vi "VisualizeDigitizer.vi"() -> ()   [LabVIEW 2014, in "Visualization.lvlib" / "VisualizeDigitizer.lvclass"]
uses:
  VisualizeDigitizer.lvclass
  Digitizer/DigitizerPlugins/DigitizerBaseClass/Typedefs/WfrmAttributes.ctl
  VisualizeBase/VisualizeBase_class/Requests/clUserEventType.ctl
  <vilib>/event_ctls.llb/usereventprio.ctl
  <vilib>/Utility/error.llb/Error Cluster From Error Code.vi
  <vilib>/ErrorRing/Error Ring.xnode
  VisualizeBase/VisualizeBase_class/VisualizeBase.lvclass
  <userlib>/NIST/NISTErrorLib/NISTErrorLib.lvlib
  Digitizer/DigitizerModule/DigitizerModule.lvlib
  Digitizer/DigitizerPlugins/DigitizerBaseClass/DigitizerBase.lvclass
panel:
  out "Timing":cluster{"Time Stamp":timestamp, "dt":dbl}[][](array[cluster])
  in  "btnReset":bool
  in  "btnClear":bool
  out "Attributes":T1[][](array[typedef])
  out "Waveform":waveform(dbl)[](graph)
  in  "QueName":string="DigitizerVisQue"
  out "ErrorArray":errorcluster[](array[cluster])
  in  "btnStop":bool
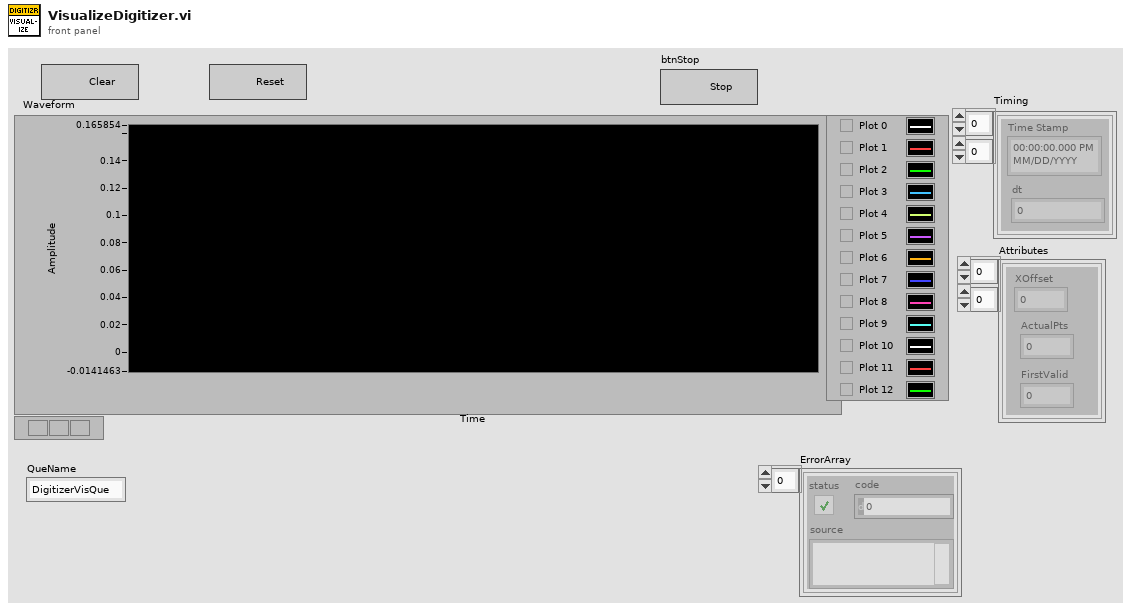
[diagram p1: front panel]
types:
  T1 = typedef "DigitizerPlugins.lvlib/DigitizerBase.lvclass/WfrmAttributes.ctl" = cluster{"XOffset":dbl, "ActualPts":i64, "FirstValid":i64}
  T2 = typedef "Visualization.lvlib/VisualizeBase.lvclass/clRequestEvents.ctl" = cluster{"StopRequest":refnum<user-event>, "ResetRequest":refnum<user-event>}
  T3 = typedef "DigitizerModule.lvlib/clBroadcastEvents.ctl" = cluster{"DidInit":refnum<user-event>, "StatusUpdate":refnum<user-event>, "ErrorReport":refnum<user-event>, "DidStop":refnum<user-event>, "PathToINI":refnum<user-event>, "Channels":refnum<user-event>, "Acq":refnum<user-event>, "Trigger":refnum<user-event>, "Waveforms":refnum<user-event>}
  T4 = typedef "Visualization.lvlib/VisualizeBase.lvclass/clUserEventType.ctl" = cluster{"BusIndex":i8, "Data":variant}
  T5 = typedef "usereventprio.ctl" = enum32{"high priority", "normal priority"}
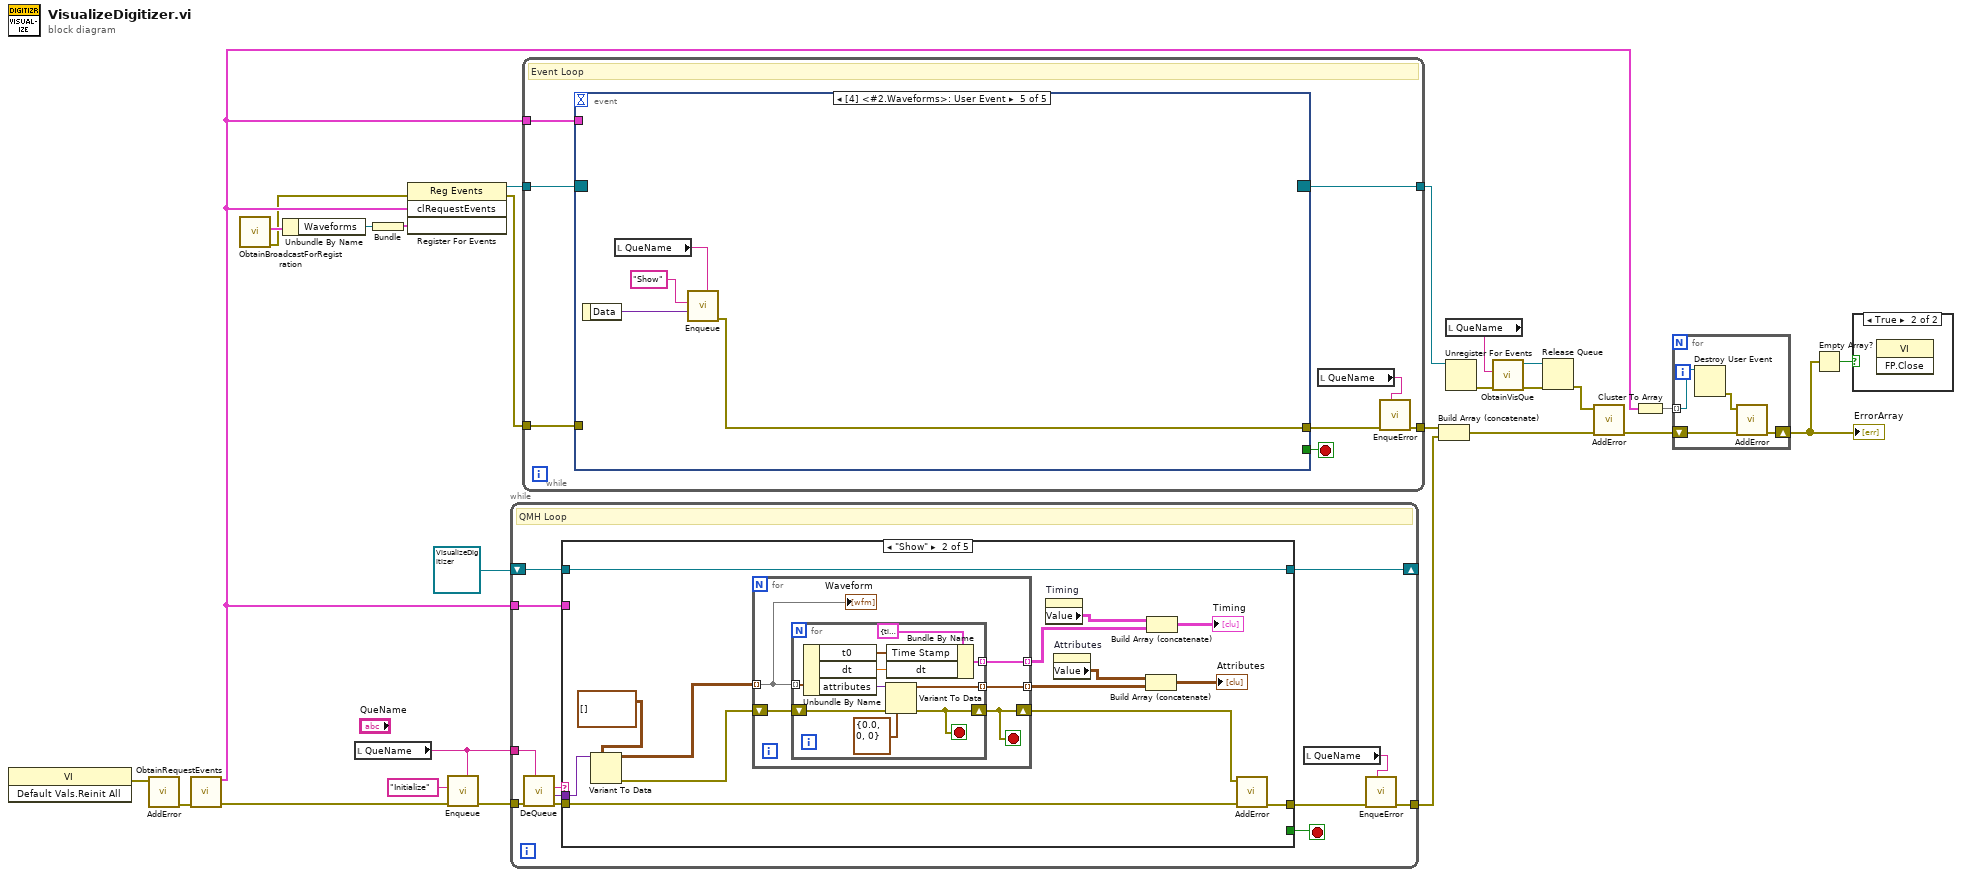
[diagram p0: block diagram]
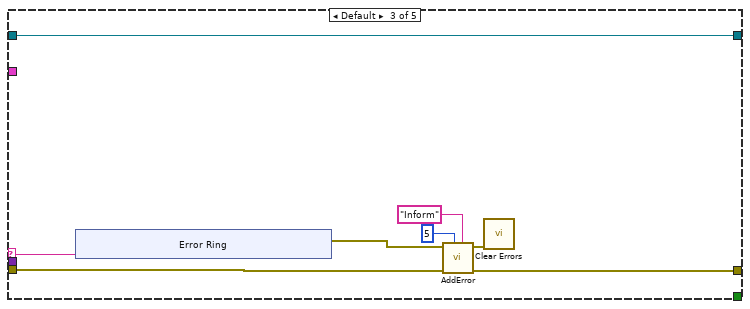
[diagram p4: hidden frame]
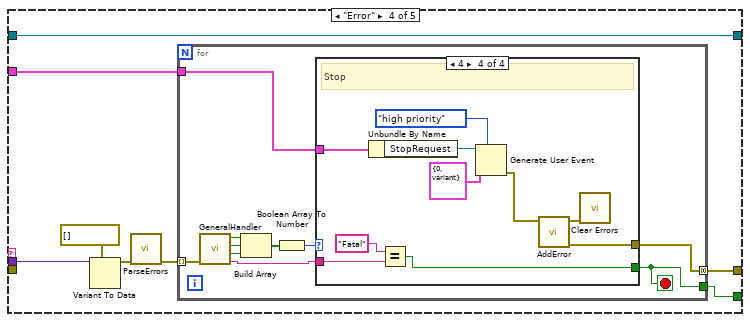
[diagram p5: hidden frame]
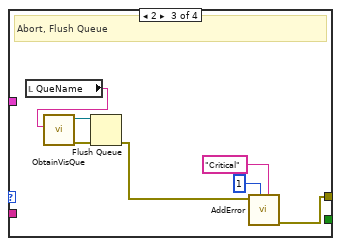
[diagram p8: hidden frame]
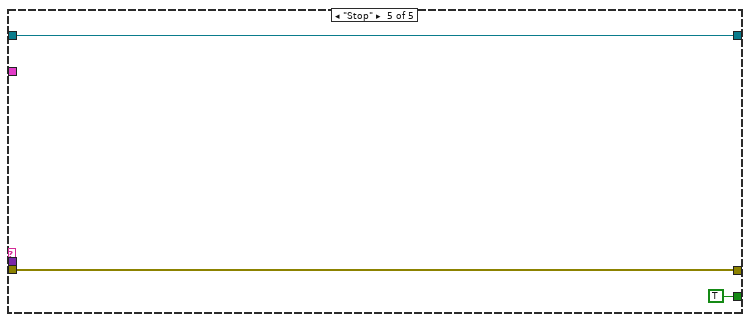
[diagram p9: hidden frame]
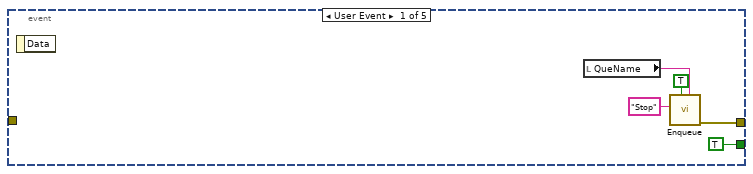
[diagram p10: hidden frame]
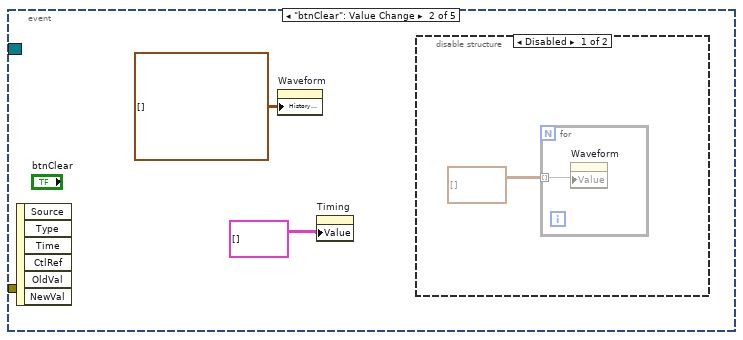
[diagram p11: hidden frame]
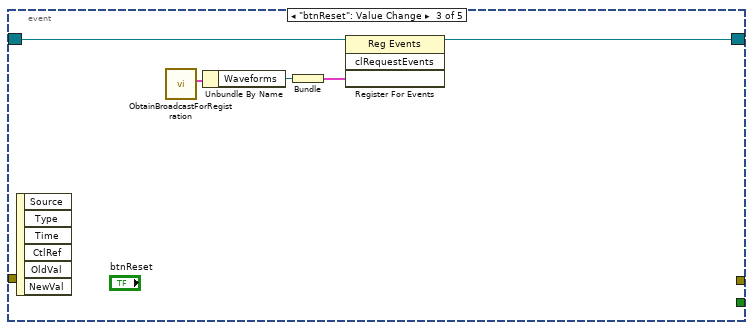
[diagram p13: hidden frame]
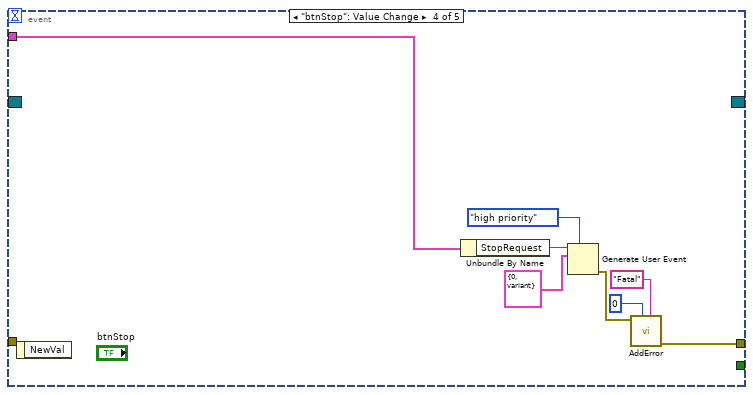
[diagram p14: hidden frame]
diagram:
  n1 = invoke class="VI" method="Default Vals.Reinit All"() -> (error out=w24:errorcluster)  [unwired: 3 in, 2 out]
  n2 = call <userlib>:"AddError.vi"("error in (no error)"=w24) -> ("ErrorArray"=w23:errorcluster[])  [unwired: 9 in, 1 out]
  n3 = call "ObtainRequestEvents.vi"("Error"=w23) -> ("Error"=w3:errorcluster[], "clRequestEvents"=w9:T2)  [unwired: 9 in]
  n4 = call "ObtainBroadcastForRegistration.vi"() -> ("error out"=w2:errorcluster, "clDigitizerBdcstEvents"=w6:T3)  [unwired: 10 in]
  n5 = Unbundle By Name(w6) -> ("Waveforms"=w5:refnum<user-event>)
  n6 = local read "QueName"() -> (w22:string)
  n7 = Bundle("Waveforms"=w5) -> (w4:cluster{"Waveforms":refnum<user-event>})  [unwired: 1 in]
  n8 = register-events(error in=w2, w9, w4) -> (reference out=w25:refnum<event-registration>, error out=w1:errorcluster)  [unwired: 1 in]
  n9 = call "Enqueue.vi"("QueName"=w22, "Error"=w3, "Message"="Initialize") -> ("Error"=w26:errorcluster[])  [unwired: 8 in]
  n10 = while {
    tunnel: w26 -> [w39]
    tunnel: [w33] -> w17
    tunnel: w22 -> [w31]
    shift-right: [w30] -> _
    shift-left: refnum<class "VisualizeDigitizer.lvclass"> refnum ("VisualizeBase_class.lvclass") -> [w29]
    tunnel: w9 -> [w28]
    stop <- w34 stop-if-true
    # "QMH Loop"
    n11 = call "DeQueue.vi"("QueName"=w31, "Error"=w39) -> ("Error"=w36:errorcluster[], "Data"=w37:variant, "Message"=w38:string)  [unwired: 7 in]
    n12 = case shown="\"Show\"" w38 {
      selector: w38 -> [_ _ w78 _ _]
      tunnel: w37 -> [_ w55 _ w93 _]
      tunnel: w36 -> [w41 w51 w76 _ w122]
      tunnel: [w41 w52 w75 w89 w122] -> w35
      tunnel: [_ _ _ w88 TRUE] -> w34
      tunnel: w29 -> [w40 w50 w71 w87 w121]
      tunnel: [w40 w50 w71 w87 w121] -> w30
      tunnel: w28 -> [_ _ _ w86 _]
      frame "Initialize" {
      }
      frame "Show" {
        n13 = Variant To Data(type=waveform(dbl)[][] [] ("data"), Variant=w55) -> (data=w42:waveform(dbl)[][], error out=w44:errorcluster)  [unwired: 1 in]
        n14 = for {
          tunnel: w42 -> [w59] mode=indexing
          tunnel: [w60] -> w53 mode=indexing
          tunnel: [w58] -> w48 mode=indexing
          shift-right: [w56] -> w43
          shift-left: w44 -> [w57]
          stop <- w56 stop-if-true
          n15 = for {
            tunnel: w59 -> [w70] mode=indexing
            tunnel: [w67] -> w60 mode=indexing
            tunnel: [w63] -> w58 mode=indexing
            shift-right: [w61] -> w56
            shift-left: w57 -> [w62]
            stop <- w61 stop-if-true
            n16 = Unbundle By Name(w70) -> ("t0"=w65:timestamp, "dt"=w64:dbl, "attributes"=w69:variant)
            n17 = Variant To Data(error in=w62, type=T1 {"XOffset"=0.0, "ActualPts"=0, "FirstValid"=0} ("Attributes"), Variant=w69) -> (data=w67:T1, error out=w61:errorcluster)
            n18 = Bundle By Name(cluster=cluster{"Time Stamp":timestamp, "dt":dbl} {"Time Stamp"=timestamp(0 s since 1904-01-01), "dt"=0.0} ("Cluster"), "Time Stamp"=w65, "dt"=w64) -> (w63:cluster{"Time Stamp":timestamp, "dt":dbl})
          }
          "Waveform" <- w59
        }
        n19 = property on="Timing" class="Arr (strict)"() -> ("Value"=w49:cluster{"Time Stamp":timestamp, "dt":dbl}[][])  [unwired: 2 in, 2 out]
        n20 = property on="Attributes" class="Arr (strict)"() -> ("Value"=w45:T1[][])  [unwired: 2 in, 2 out]
        n21 = Build Array (concatenate)(w45, w53) -> (→"Attributes":T1[][])
        n22 = Build Array (concatenate)(w49, w48) -> (→"Timing":cluster{"Time Stamp":timestamp, "dt":dbl}[][])
        n23 = call <userlib>:"AddError.vi"("ErrorArray"=w51, "error in (no error)"=w43) -> ("ErrorArray"=w52:errorcluster[])  [unwired: 8 in, 1 out]
      }
      frame Default {
        n24 = xnode "Error Ring"("parameter 0"=w78) -> ("error out"=w77:errorcluster)
        n25 = call <userlib>:"AddError.vi"("Severity"="Inform" ("String"), "Priority"=u8 5, "ErrorArray"=w76, "error in (no error)"=w77) -> ("ErrorArray"=w75:errorcluster[], "error out"=w74:errorcluster)  [unwired: 6 in]
        n26 = call <vilib>:"Clear Errors.vi"("error in (no error)"=w74) -> ()  [unwired: 5 in, 2 out]
      }
      frame "Error" {
        n27 = Variant To Data(type=errorcluster[] [], Variant=w93) -> (data=w91:errorcluster[])  [unwired: 1 in, 1 out]
        n28 = call <userlib>:"ParseErrors.vi"("ErrorArray"=w91) -> ("ErrorArray"=w90:errorcluster[])  [unwired: 8 in, 2 out]
        n29 = for {
          tunnel: w90 -> [w103] mode=indexing
          tunnel: [w97] -> w89 mode=concatenating
          tunnel: [w95] -> w88
          tunnel: w86 -> [w94]
          stop <- w95 stop-if-true
          n30 = call <userlib>:"GeneralHandler.vi"("error in (no error)"=w103) -> ("Severity"=w96:string, "Stop"=w100:bool, "Abort"=w101:bool, "Continue"=w102:bool)  [unwired: 7 in]
          n31 = Build Array(w102, w101, w100) -> (w99:bool[])
          n32 = Boolean Array To Number(Boolean array=w99) -> (number=w98:u32)
          n33 = case shown="4" w98 {
            tunnel: [_ _ w108 w119] -> w97
            tunnel: w96 -> [_ _ _ w114]
            tunnel: [_ _ _ w112] -> w95
            tunnel: w94 -> [_ _ _ w111]
            frame 0, Default {
              # "No Dialog"
            }
            frame 1 {
              # "Continue"
            }
            frame 2 {
              # "Abort, Flush Queue"
              n34 = local read "QueName"() -> (w104:string)
              n35 = call "ObtainVisQue.vi"("QueName"=w104) -> ("error out"=w110:errorcluster, "queue out"=w109:refnum<queue>)  [unwired: 9 in]
              n36 = Flush Queue(queue=w109, error in (no error)=w110) -> (error out=w107:errorcluster)  [unwired: 2 out]
              n37 = call <userlib>:"AddError.vi"("Severity"="Critical" ("String"), "Priority"=u8 1, "error in (no error)"=w107) -> ("ErrorArray"=w108:errorcluster[])  [unwired: 7 in, 1 out]
            }
            frame 4 {
              # "Stop"
              n38 = Unbundle By Name(w111) -> ("StopRequest"=w120:refnum<user-event>)
              n39 = Equal?(x="Fatal", y=w114) -> (x = y?=w112:bool)
              n40 = Generate User Event(priority (normal)=usereventprio."high priority", user event=w120, event data cluster=T4 {"BusIndex"=0, "Data"=variant} ("event data")) -> (error out=w118:errorcluster)  [unwired: 1 in, 1 out]
              n41 = call <userlib>:"AddError.vi"("error in (no error)"=w118) -> ("ErrorArray"=w119:errorcluster[], "error out"=w115:errorcluster)  [unwired: 9 in]
              n42 = call <vilib>:"Clear Errors.vi"("error in (no error)"=w115) -> ()  [unwired: 5 in, 2 out]
            }
          }
        }
      }
      frame "Stop" {
      }
    }
    n43 = local read "QueName"() -> (w32:string)
    n44 = call "EnqueError.vi"("QueName"=w32, "Error"=w35) -> ("Error"=w33:errorcluster[])  [unwired: 9 in]
  }
  n45 = while {
    tunnel: w25 -> [w131]
    tunnel: [w128] -> w18
    tunnel: [w126] -> w20
    tunnel: w9 -> [w125]
    tunnel: w1 -> [w124]
    stop <- w130 stop-if-true
    # "Event Loop"
    n46 = event shown="[4] <#2.Waveforms>: User Event" {
      selector: w131 -> [_ _ w145 _ _]
      dyn-events: [_ _ w144 _ _] -> w126
      timeout: _ -> [_ _ _ _ _]
      tunnel: [TRUE _ _ _ _] -> w130
      tunnel: [w135 _ _ w151 w155] -> w129
      tunnel: w125 -> [_ _ _ w146 _]
      tunnel: w124 -> [_ _ _ _ _]
      event User Event {
        n47 = event-data() -> ()  [unwired: 1 in, 1 out]
        n48 = local read "QueName"() -> (w132:string)
        n49 = call "Enqueue.vi"("QueName"=w132, "Priority? (F)"=TRUE, "Message"="Stop") -> ("Error"=w135:errorcluster[])  [unwired: 8 in]
      }
      event "btnClear": Value Change {
        n50 = event-data() -> ()  [unwired: 1 in, 6 out]
        n51 = property on="Waveform" class="WFChart (strict)"("History Data"=waveform(dbl)[][] []) -> ()  [unwired: 2 in, 2 out]
        n52 = property on="Timing" class="Arr (strict)"("Value"=cluster{"Time Stamp":timestamp, "dt":dbl}[][] [] ("Timing")) -> ()  [unwired: 2 in, 2 out]
        n53 = disable-structure shown="Disabled" {
          frame Disabled {
            n54 = for {
              tunnel: waveform(dbl)[][] [] ("Waveform Graph") -> [w140] mode=indexing
              n55 = property on="Waveform" class="WFChart (strict)"("Value"=w140) -> ()  [unwired: 2 in, 2 out]
            }
          }
          frame Enabled {
          }
        }
      }
      event "btnReset": Value Change {
        n56 = event-data() -> ()  [unwired: 1 in, 6 out]
        n57 = call "ObtainBroadcastForRegistration.vi"() -> ("clDigitizerBdcstEvents"=w142:T3)  [unwired: 10 in, 1 out]
        n58 = Unbundle By Name(w142) -> ("Waveforms"=w143:refnum<user-event>)
        n59 = Bundle("Waveforms"=w143) -> (w141:cluster{"Waveforms":refnum<user-event>})  [unwired: 1 in]
        n60 = register-events(reference=w145, w141) -> (reference out=w144:refnum<event-registration>)  [unwired: 2 in, 1 out]
      }
      event "btnStop": Value Change {
        n61 = event-data() -> ()  [unwired: 1 in, 1 out]
        n62 = Unbundle By Name(w146) -> ("StopRequest"=w152:refnum<user-event>)
        n63 = Generate User Event(priority (normal)=usereventprio."high priority", user event=w152, event data cluster=T4 {"BusIndex"=0, "Data"=variant} ("event data")) -> (error out=w153:errorcluster)  [unwired: 1 in, 1 out]
        n64 = call <userlib>:"AddError.vi"("Severity"="Fatal" ("String"), "Priority"=u8 0, "error in (no error)"=w153) -> ("ErrorArray"=w151:errorcluster[])  [unwired: 7 in, 1 out]
      }
      event User Event {
        n65 = event-data() -> ("Data"=w157:variant)  [unwired: 1 in]
        n66 = local read "QueName"() -> (w154:string)
        n67 = call "Enqueue.vi"("QueName"=w154, "Data"=w157, "Message"="Show") -> ("Error"=w155:errorcluster[])  [unwired: 8 in]
      }
    }
    n68 = local read "QueName"() -> (w127:string)
    n69 = call "EnqueError.vi"("QueName"=w127, "Error"=w129) -> ("Error"=w128:errorcluster[])  [unwired: 9 in]
  }
  n70 = Build Array (concatenate)(w18, w17) -> (w14:errorcluster[])
  n71 = local read "QueName"() -> (w15:string)
  n72 = Unregister For Events(event registration refnum=w20) -> (error out=w16:errorcluster)  [unwired: 1 in]
  n73 = call "ObtainVisQue.vi"("error in (no error)"=w16, "QueName"=w15) -> ("error out"=w13:errorcluster, "queue out"=w12:refnum<queue>)  [unwired: 8 in]
  n74 = Release Queue(queue=w12, error in (no error)=w13) -> (error out=w11:errorcluster)  [unwired: 1 in, 2 out]
  n75 = call <userlib>:"AddError.vi"("ErrorArray"=w14, "error in (no error)"=w11) -> ("ErrorArray"=w10:errorcluster[])  [unwired: 8 in, 1 out]
  n76 = Cluster To Array(cluster=w9) -> (array=w19:refnum<user-event>[])
  n77 = for {
    tunnel: w19 -> [w161] mode=indexing
    shift-right: [w160] -> w8
    shift-left: w10 -> [w159]
    n78 = Destroy User Event(user event=w161) -> (error out=w158:errorcluster)  [unwired: 1 in]
    n79 = call <userlib>:"AddError.vi"("ErrorArray"=w159, "error in (no error)"=w158) -> ("ErrorArray"=w160:errorcluster[])  [unwired: 8 in, 1 out]
  }
  "ErrorArray" <- w8
  n80 = Empty Array?(array=w8) -> (empty?=w7:bool)
  n81 = case shown="True" w7 {
    frame False {
    }
    frame True {
      n82 = invoke class="VI" method="FP.Close"() -> ()  [unwired: 3 in, 3 out]
    }
  }
